vi "AppPath Check.vi"(8 "error in (no error)":errorcluster, 11 "Controller in":refnum<class "Controller.lvclass">) -> (0 "error out":errorcluster, 2 "App Folder":path, 3 "Controller out":refnum<class "Controller.lvclass">)   [LabVIEW 2020, in "Controller.lvlib" / "Controller.lvclass"]
uses:
  Controller.lvclass
  <vilib>/Utility/sysdir.llb/System Directory Type.ctl
  Controller.lvclass/Controller.ctl
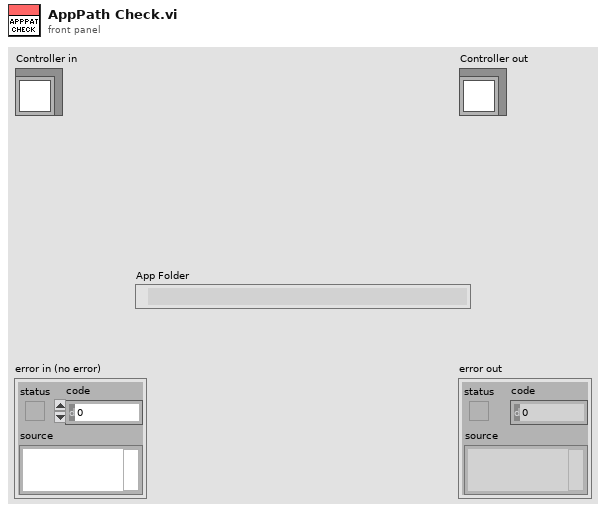
[diagram p1: front panel]
types:
  T1 = enum16{"open", "replace", "create", "open or create", "replace or create", "replace or create with confirmation"}
  T2 = typedef "System Directory Type.ctl" = i32
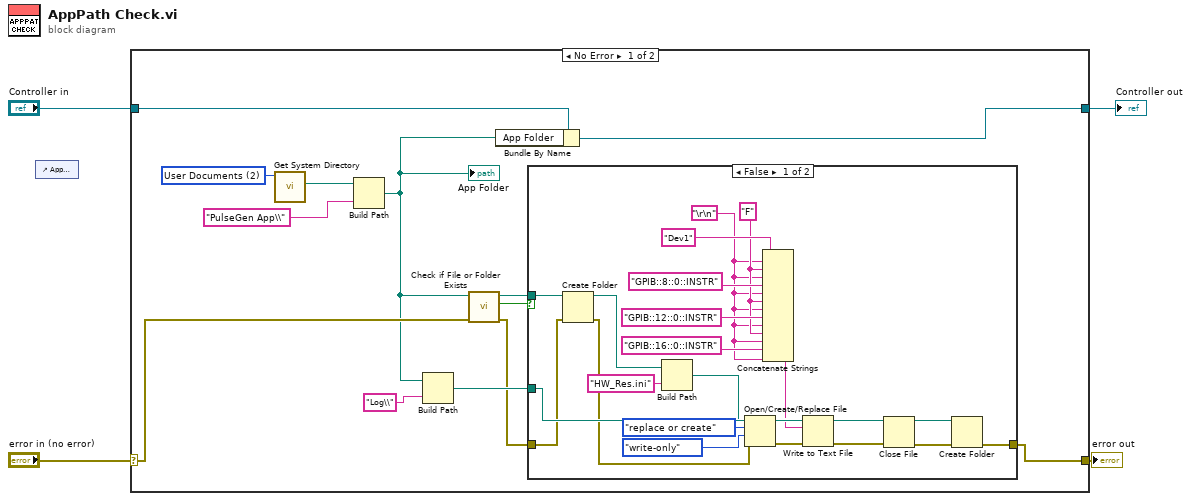
[diagram p0: block diagram]
diagram:
  n1 = control-ref of="App Folder"() -> ()  [unwired: 1 out]
  n2 = case shown="No Error" "error in (no error)" {
    selector: "error in (no error)" -> [w10 w42]
    tunnel: [w8 w42] -> w3
    tunnel: [w5 w41] -> w1
    tunnel: "Controller in" -> [w7 w41]
    frame No Error {
      w11 = T2 2 items=["User Home", "User Desktop", "User Documents", "User Application Data", "User Preferences", "User Temporary", "Public Documents", "Public Application Data", "Public Preferences", "System Core Libraries", "System Installed Libraries", "Application Files", "Boot Volume Root"] ("system directory type")
      n3 = call <vilib>:"Get System Directory.vi"("system directory type"=w11) -> ("system directory"=w12:path)  [unwired: 10 in]
      n4 = Build Path(base path=w12, name or relative path="PulseGen App\\") -> (appended path=w6:path)
      "App Folder" <- w6
      n5 = Build Path(base path=w6, name or relative path="Log\\") -> (appended path=w17:path)
      n6 = call <vilib>:"Check if File or Folder Exists.vi"("error in (no error)"=w10, "path"=w6) -> ("error out"=w9:errorcluster, "file or folder exists?"=w14:bool, "dup path"=w15:path)  [unwired: 7 in]
      n7 = Bundle By Name(cluster=w7, "App Folder"=w6) -> (w5:refnum<class "Controller.lvclass">)
      n8 = case shown="False" w14 {
        tunnel: w15 -> [w39 _]
        tunnel: w17 -> [w38 _]
        tunnel: w9 -> [w37 w40]
        tunnel: [w36 w40] -> w8
        frame False {
          w19 = "F" ("string")
          w18 = "\r\n"
          n9 = Create Folder(path (use dialog)=w39, error in=w37) -> (created path=w25:path, error out=w26:errorcluster)  [unwired: 1 in, 1 out]
          n10 = Build Path(base path=w25, name or relative path="HW_Res.ini") -> (appended path=w31:path)
          n11 = Open/Create/Replace File(file path (use dialog)=w31, error in=w26, operation (0:open)=T1."replace or create", access (0:read/write)=enum16{"read/write", "read-only", "write-only"}."write-only") -> (refnum out=w33:refnum<file>, error out=w32:errorcluster)  [unwired: 2 in, 1 out]
          n12 = Concatenate Strings("Dev1" ("string"), w18, w19, w18, "GPIB::8::0::INSTR" ("string"), w18, w19, w18, "GPIB::12::0::INSTR" ("string"), w18, w19, w18, "GPIB::16::0::INSTR" ("string"), w18) -> (w20:string)
          n13 = Write to Text File(file (use dialog)=w33, text=w20, error in=w32) -> (refnum out=w35:refnum<file>, error out=w34:errorcluster)  [unwired: 1 in, 1 out]
          n14 = Close File(refnum=w35, error in=w34) -> (error out=w27:errorcluster)  [unwired: 1 out]
          n15 = Create Folder(path (use dialog)=w38, error in=w27) -> (error out=w36:errorcluster)  [unwired: 1 in, 2 out]
        }
        frame True {
        }
      }
    }
    frame Error {
    }
  }
  "error out" <- w3
  "Controller out" <- w1
